vi "tc_selection_new.vi"(10 "Coords":T1, 11 "Position":T2) -> (3 "Numeric":i32)   [LabVIEW 2016]
uses:
  <vilib>/Utility/miscctls.llb/LVPositionTypeDef.ctl
  <vilib>/Utility/miscctls.llb/LVPoint32TypeDef.ctl
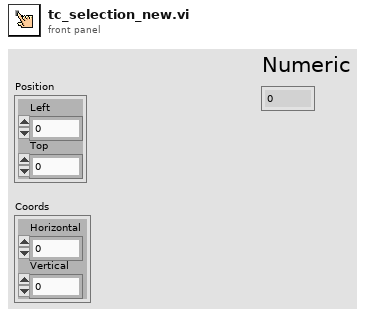
[diagram p1: front panel]
types:
  T1 = typedef "LVPoint32TypeDef.ctl" = cluster{"Horizontal":i32, "Vertical":i32}
  T2 = typedef "LVPositionTypeDef.ctl" = cluster{"Left":i32, "Top":i32}
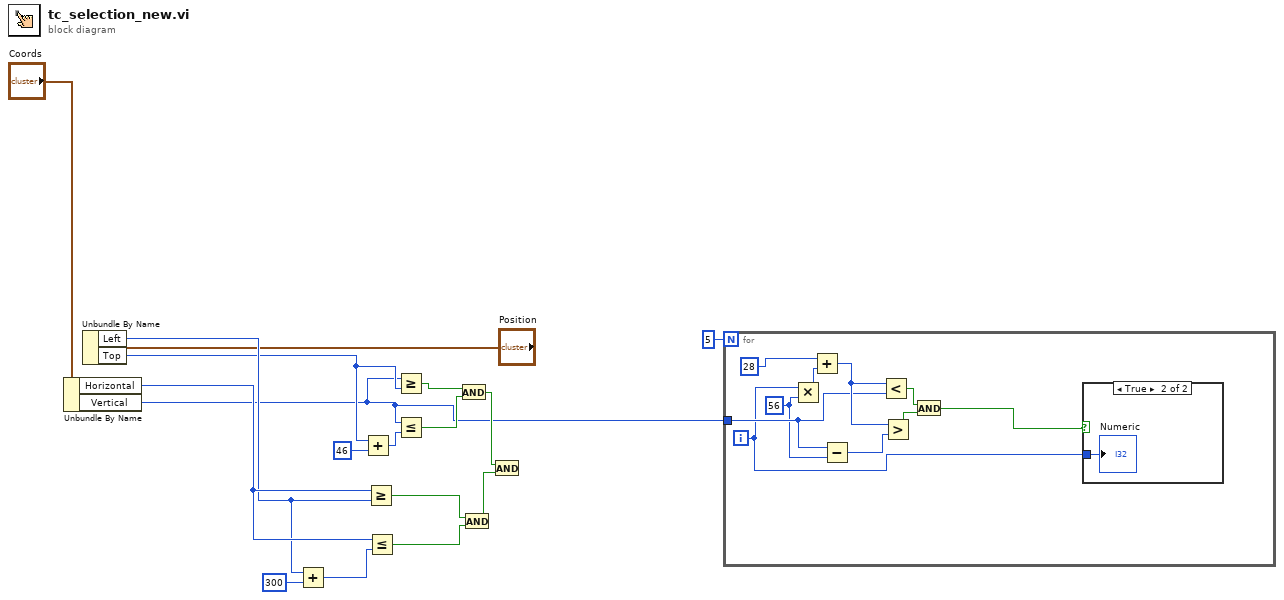
[diagram p0: block diagram]
diagram:
  n1 = Unbundle By Name("Coords") -> ("Horizontal"=w14:i32, "Vertical"=w1:i32)
  n2 = Unbundle By Name("Position") -> ("Left"=w11:i32, "Top"=w9:i32)
  n3 = Add(x=w11, y=300) -> (x+y=w12:i32)
  n4 = Add(x=w9, y=46) -> (x+y=w8:i32)
  n5 = Greater Or Equal?(x=w14, y=w11) -> (x >= y?=w10:bool)
  n6 = Less Or Equal?(x=w14, y=w12) -> (x <= y?=w15:bool)
  n7 = Greater Or Equal?(x=w1, y=w9) -> (x >= y?=w5:bool)
  n8 = Less Or Equal?(x=w1, y=w8) -> (x <= y?=w6:bool)
  n9 = And(x=w5, y=w6) -> (x .and. y?=w17:bool)
  n10 = And(x=w10, y=w15) -> (x .and. y?=w16:bool)
  n11 = And(x=w17, y=w16) -> ()  [unwired: 1 out]
  n12 = for {
    N: 5 -> [_]
    tunnel: w1 -> [w23]
    i -> [w18]
    w22 = 56
    n13 = Multiply(x=w18, y=w22) -> (x*y=w27:i32)
    n14 = Add(x=28, y=w27) -> (x+y=w25:i32)
    n15 = Subtract(x=w23, y=w22) -> (x-y=w24:i32)
    n16 = Less?(x=w25, y=w23) -> (x < y?=w20:bool)
    n17 = Greater?(x=w25, y=w24) -> (0:w21:bool)
    n18 = And(x=w20, y=w21) -> (x .and. y?=w19:bool)
    n19 = case shown="True" w19 {
      tunnel: w18 -> [_ w28]
      frame False {
      }
      frame True {
        "Numeric" <- w28
      }
    }
  }
